vi "PRIME Telescope Convert RA and DEC to HHMMSS.vi"(11 "RA and DEC":T3) -> (0 "Dec String":string, 1 "RA String":string, 2 "Declination":T1, 3 "Right Ascension":T2)   [LabVIEW 2024, in "PRIME Telescope.lvclass"]
uses:
  PRIME Telescope.lvclass
  typedefs/CC cluster RA and DEC.ctl
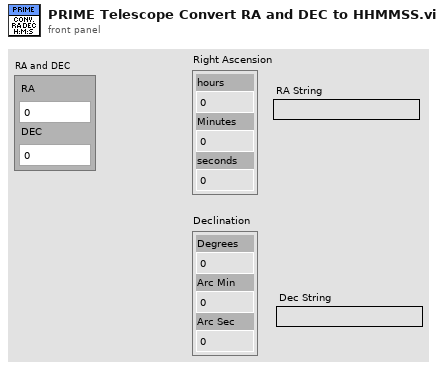
[diagram p1: front panel]
types:
  T1 = cluster{"Degrees":dbl, "Arc Min":dbl, "Arc Sec":dbl}
  T2 = cluster{"hours":dbl, "Minutes":dbl, "seconds":dbl}
  T3 = typedef "CC cluster RA and DEC.ctl" = cluster{"RA":dbl, "DEC":dbl}
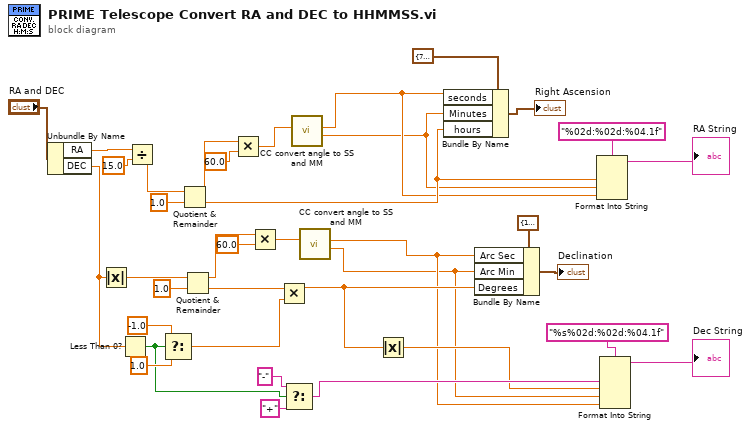
[diagram p0: block diagram]
diagram:
  n1 = Unbundle By Name("RA and DEC") -> ("RA"=w35:dbl, "DEC"=w18:dbl)
  n2 = Absolute Value(x=w18) -> (abs(x)=w19:dbl)
  n3 = Less Than 0?(x=w18) -> (x < 0?=w10:bool)
  n4 = Divide(x=w35, y=15.0) -> (x/y=w33:dbl)
  n5 = Select(t=-1.0, s=w10, f=1.0) -> (s? t:f=w15:dbl)
  n6 = Quotient & Remainder(x=w33, y=1.0) -> (x-y*floor(x/y)=w31:dbl, floor(x/y)=w21:dbl)
  n7 = Quotient & Remainder(x=w19, y=1.0) -> (x-y*floor(x/y)=w27:dbl, floor(x/y)=w24:dbl)
  n8 = Multiply(x=w31, y=60.0) -> (x*y=w6:dbl)
  n9 = Multiply(x=w27, y=60.0) -> (x*y=w3:dbl)
  n10 = Multiply(x=w24, y=w15) -> (x*y=w8:dbl)
  n11 = Select(t="-", s=w10, f="+") -> (s? t:f=w9:string)
  n12 = call "CC convert angle to SS and MM.vi"("Angle"=w6) -> ("Minutes"=w4:dbl, "Seconds"=w5:dbl)  [unwired: 9 in]
  n13 = call "CC convert angle to SS and MM.vi"("Angle"=w3) -> ("Minutes"=w1:dbl, "Seconds"=w2:dbl)  [unwired: 9 in]
  n14 = Absolute Value(x=w8) -> (abs(x)=w7:dbl)
  n15 = Bundle By Name(cluster=T2 {"hours"=7.0, "Minutes"=57.0, "seconds"=16.79999999999879} ("Degrees"), "seconds"=w5, "Minutes"=w4, "hours"=w21) -> (→"Right Ascension":T2)
  n16 = Bundle By Name(cluster=T1 {"Degrees"=10.0, "Arc Min"=2.0, "Arc Sec"=11.040000000001555} ("Declination"), "Arc Sec"=w2, "Arc Min"=w1, "Degrees"=w8) -> (→"Declination":T1)
  n17 = Format Into String(format string="%02d:%02d:%04.1f", w21, w4, w5) -> (resulting string=→"RA String":string)  [unwired: 2 in, 1 out]
  n18 = Format Into String(format string="%s%02d:%02d:%04.1f", w9, w7, w1, w2) -> (resulting string=→"Dec String":string)  [unwired: 2 in, 1 out]
